vi "Channel 0 Initiate Start Up (SubVI).vi"(10 "Channel # in":i32, 11 "VISA Refnum in":refnum<visa-resource-name>) -> (0 "error out":errorcluster, 2 "BoardHandle out":T1)   [LabVIEW 2020]
uses:
  SUB VI Dark Current Test Files 2018 For Drop Box/Program Files (x86)/National Instruments/LabVIEW 2020/instr.lib/CAEN PSM/CAEN PSM.lvlib
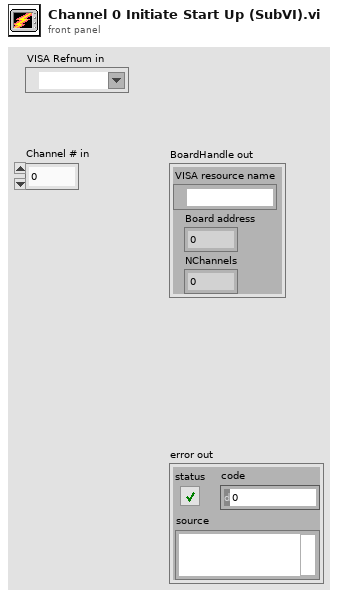
[diagram p1: front panel]
types:
  T1 = cluster{"VISA resource name":refnum<visa-resource-name>, "Board address":u8, "NChannels":u8}
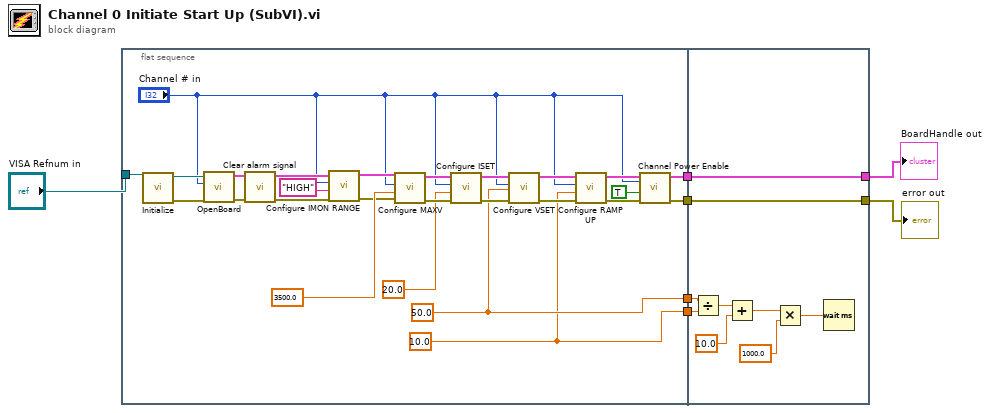
[diagram p0: block diagram]
diagram:
  n1 = flat-sequence {
    tunnel: [w19] -> w7
    tunnel: [w18] -> w6
    tunnel: [w17] -> w5
    tunnel: [w16] -> w4
    tunnel: "VISA Refnum in" -> [w15]
    tunnel: w7 -> [w37]
    tunnel: w6 -> [w36]
    tunnel: [w35] -> w3
    tunnel: w5 -> [w35]
    tunnel: [w34] -> w2
    tunnel: w4 -> [w34]
    frame #0 {
      w19 = 50.0 ("Voltage Set (Volts)")
      w18 = 10.0 ("Voltage Ramp Up (V/s)")
      n2 = call "Initialize.vi"("VISA resource name"=w15) -> ("error out"=w28:errorcluster, "VISA resource name out"=w25:refnum<visa-resource-name>)  [unwired: 9 in]
      n3 = call "OpenBoard.vi"("error in (no error)"=w28, "Board Address"="Channel # in", "VISA resource name"=w25) -> ("error out"=w29:errorcluster, "BoardHandle"=w24:T1)  [unwired: 7 in]
      n4 = call "Clear alarm signal.vi"("error in (no error)"=w29, "BoardHandle"=w24) -> ("error out"=w13:errorcluster, "BoardHandle out"=w12:T1)  [unwired: 8 in]
      n5 = call "Configure IMON RANGE.vi"("error in (no error)"=w13, "IMon range (LOW)"="HIGH", "Channel (0)"="Channel # in", "BoardHandle"=w12) -> ("error out"=w9:errorcluster, "BoardHandle out"=w10:T1)  [unwired: 6 in]
      n6 = call "Configure MAXV.vi"("error in (no error)"=w9, "Voltage Max (0.0 V)"=3500.0 ("VMax (Volts)"), "Channel (0)"="Channel # in", "BoardHandle"=w10) -> ("error out"=w30:errorcluster, "BoardHandle out"=w23:T1)  [unwired: 6 in]
      n7 = call "Configure ISET.vi"("error in (no error)"=w30, "Current Limit (0.00 uA)"=20.0 ("Current Limit (uA)"), "Channel (0)"="Channel # in", "BoardHandle"=w23) -> ("error out"=w31:errorcluster, "BoardHandle out"=w22:T1)  [unwired: 6 in]
      n8 = call "Configure VSET.vi"("error in (no error)"=w31, "Voltage Level (0.0 V)"=w19, "Channel (0)"="Channel # in", "BoardHandle"=w22) -> ("error out"=w32:errorcluster, "BoardHandle out"=w21:T1)  [unwired: 6 in]
      n9 = call "Configure RAMP UP.vi"("error in (no error)"=w32, "Voltage ramp up (0 V/s)"=w18, "Channel (0)"="Channel # in", "BoardHandle"=w21) -> ("error out"=w33:errorcluster, "BoardHandle out"=w20:T1)  [unwired: 6 in]
      n10 = call "Channel Power Enable.vi"("error in (no error)"=w33, "Enable (OFF)"=TRUE ("Boolean"), "Channel (0)"="Channel # in", "BoardHandle"=w20) -> ("error out"=w16:errorcluster, "BoardHandle out"=w17:T1)  [unwired: 6 in]
    }
    frame #1 {
      n11 = Divide(x=w37, y=w36) -> (x/y=w40:dbl)
      n12 = Add(x=w40, y=10.0) -> (x+y=w41:dbl)
      n13 = Multiply(x=w41, y=1000.0) -> (x*y=w42:dbl)
      n14 = Wait (ms)(milliseconds to wait=w42) -> ()  [unwired: 1 out]
    }
  }
  "BoardHandle out" <- w3
  "error out" <- w2
